vi "Controls to Commands 2017.vi"(11 "Pilot-CoPilot Controls":T6) -> (3 "All Robot Commands":T5)   [LabVIEW 2016]
uses:
  Robot Control Outputs 2017.ctl
  Drive and Climb SS/Drive + Climb Commands 2017.ctl
  Gear Delivery SS/Gear Delivery Commands.ctl
  Conveyor and Shooter SS/Conveyor and Shooter Commands.ctl
  Ball Intake SS/Ball Intake Commands.ctl
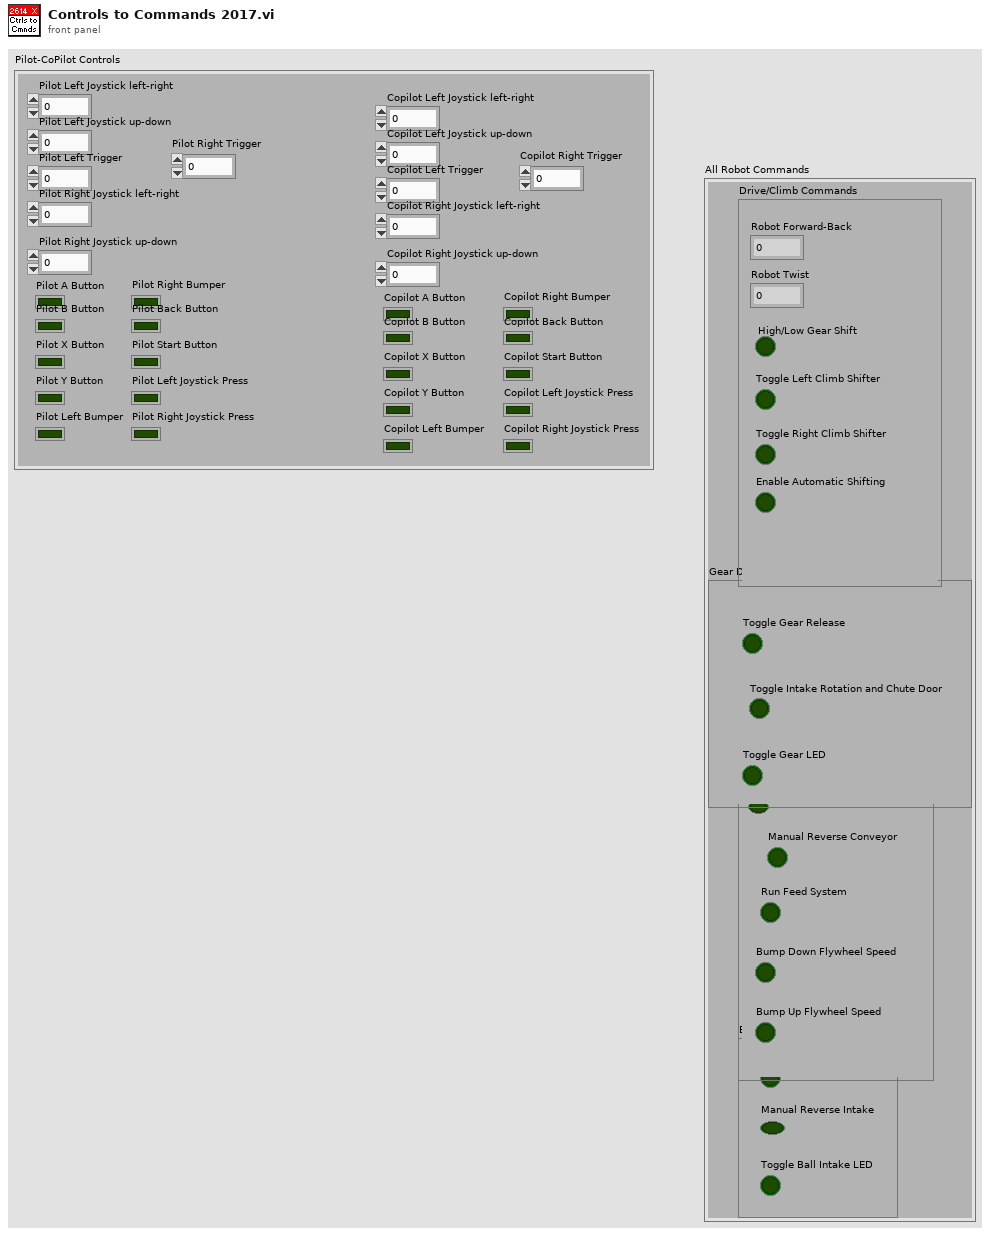
[diagram p1: front panel]
types:
  T1 = typedef "Drive + Climb Commands 2017.ctl" = cluster{"Robot Forward-Back":dbl, "Robot Twist":dbl, "High/Low Gear Shift":bool, "Toggle Left Climb Shifter":bool, "Toggle Right Climb Shifter":bool, "Enable Automatic Shifting":bool}
  T2 = typedef "Gear Delivery Commands.ctl" = cluster{"Toggle Gear Release":bool, "Toggle Intake Rotation and Chute Door":bool, "Toggle Gear LED":bool}
  T3 = typedef "Conveyor and Shooter Commands.ctl" = cluster{"Toggle Shooter":bool, "Manual Reverse Conveyor":bool, "Run Feed System":bool, "Bump Down Flywheel Speed":bool, "Bump Up Flywheel Speed":bool}
  T4 = typedef "Ball Intake Commands.ctl" = cluster{"Toggle Ball Intake":bool, "Manual Reverse Intake":bool, "Toggle Ball Intake LED":bool}
  T5 = cluster{"Drive/Climb Commands":T1, "Gear Delivery Commands":T2, "Shooter and Conveyor Commands":T3, "Ball Intake Commands":T4}
  T6 = typedef "Robot Control Outputs 2017.ctl" = cluster{"Pilot Left Joystick left-right":dbl, "Pilot Left Joystick up-down":dbl, "Pilot A Button":bool, "Pilot B Button":bool, "Pilot X Button":bool, "Pilot Y Button":bool, "Pilot Left Bumper":bool, "Pilot Right Bumper":bool, "Pilot Back Button":bool, "Pilot Start Button":bool, "Pilot Left Joystick Press":bool, "Pilot Right Joystick Press":bool, "Pilot Left Trigger":dbl, "Pilot Right Joystick left-right":dbl, "Pilot Right Joystick up-down":dbl, "Pilot Right Trigger":dbl, "Copilot Left Joystick left-right":dbl, "Copilot Left Joystick up-down":dbl, "Copilot A Button":bool, "Copilot B Button":bool, "Copilot X Button":bool, "Copilot Y Button":bool, "Copilot Left Bumper":bool, "Copilot Right Bumper":bool, "Copilot Back Button":bool, "Copilot Start Button":bool, "Copilot Left Joystick Press":bool, "Copilot Right Joystick Press":bool, "Copilot Left Trigger":dbl, "Copilot Right Joystick left-right":dbl, "Copilot Right Joystick up-down":dbl, "Copilot Right Trigger":dbl}
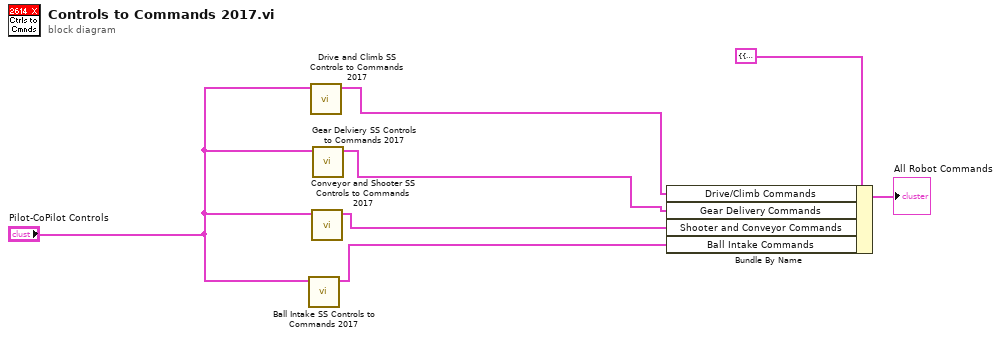
[diagram p0: block diagram]
diagram:
  n1 = call "Ball Intake SS Controls to Commands 2017.vi"("Pilot-CoPilot Controls"="Pilot-CoPilot Controls") -> ("Ball Intake Commands"=w4:T4)  [unwired: 10 in]
  n2 = call "Drive and Climb SS Controls to Commands 2017.vi"("Pilot-CoPilot Controls"="Pilot-CoPilot Controls") -> ("Drive/Climb Commands"=w2:T1)  [unwired: 10 in]
  n3 = call "Conveyor and Shooter SS Controls to Commands 2017.vi"("Pilot-CoPilot Controls"="Pilot-CoPilot Controls") -> ("Shooter and Conveyor Commands"=w3:T3)  [unwired: 10 in]
  n4 = call "Gear Delviery SS Controls to Commands 2017.vi"("Pilot-CoPilot Controls"="Pilot-CoPilot Controls") -> ("Gear Delivery Commands"=w1:T2)  [unwired: 10 in]
  n5 = Bundle By Name(cluster=T5 {"Drive/Climb Commands"={"Robot Forward-Back"=0.0, "Robot Twist"=0.0, "High/Low Gear Shift"=FALSE, "Toggle Left Climb Shifter"=FALSE, "Toggle Right Climb Shifter"=FALSE, "Enable Automatic Shifting"=FALSE}, "Gear Delivery Commands"={"Toggle Gear Release"=FALSE, "Toggle Intake Rotation and Chute Door"=FALSE, "Toggle Gear LED"=FALSE}, "Shooter and Conveyor Commands"={"Toggle Shooter"=FALSE, "Manual Reverse Conveyor"=FALSE, "Run Feed System"=FALSE, "Bump Down Flywheel Speed"=FALSE, "Bump Up Flywheel Speed"=FALSE}, "Ball Intake Commands"={"Toggle Ball Intake"=FALSE, "Manual Reverse Intake"=FALSE, "Toggle Ball Intake LED"=FALSE}} ("All Robot Commands 2"), "Drive/Climb Commands"=w2, "Gear Delivery Commands"=w1, "Shooter and Conveyor Commands"=w3, "Ball Intake Commands"=w4) -> (→"All Robot Commands":T5)
